vi "Initialize New Configuration Array.vi"(8 "error in":errorcluster, 10 "no. elements":i32, 11 "Page Refnum":refnum<vi>) -> (0 "error out":errorcluster, 3 "Page Refnum":refnum<vi>)   [LabVIEW 2014]
doc: "It writes the version number obtained from the ini file (for Push function)."
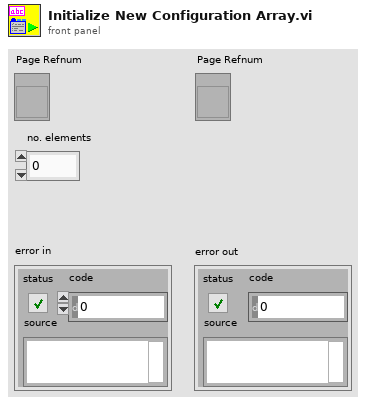
[diagram p1: front panel]
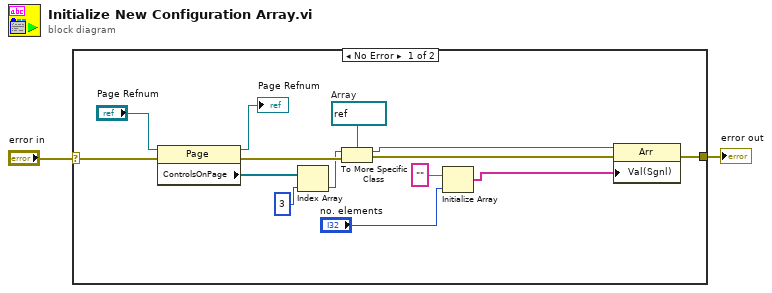
[diagram p0: block diagram]
diagram:
  n1 = case shown="No Error" "error in" {
    selector: "error in" -> [w10 w17]
    tunnel: [w8 w17] -> w2
    frame No Error {
      w12 = refnum<vi> refnum  # Array
      n2 = property class="Page"(reference="Page Refnum", error in=w10) -> (reference out=→"Page Refnum":refnum<vi>, error out=w13:errorcluster, "ControlsOnPage"=w15:refnum<vi>[])
      n3 = Index Array(array=w15, index=3) -> (element=w11:refnum<vi>)
      n4 = To More Specific Class(target class=w12, reference=w11, error in=w13) -> (specific class reference=w5:refnum<vi>, error out=w6:errorcluster)
      n5 = Initialize Array("", "no. elements") -> (w3:string[])
      n6 = property class="Arr"(reference=w5, error in=w6, "Val(Sgnl)"=w3) -> (error out=w8:errorcluster)  [unwired: 1 out]
    }
    frame Error {
    }
  }
  "error out" <- w2
